vi "Chk_cre_dir.vi"(2 "error in (no error)":errorcluster, 3 "Path":path) -> (0 "error out":errorcluster, 1 "dup path":path)   [LabVIEW 2020]
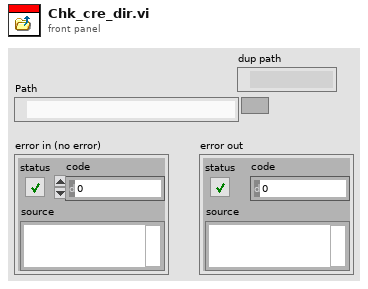
[diagram p1: front panel]
types:
  T1 = enum16{"open", "replace", "create", "open or create", "replace or create", "replace or create with confirmation"}
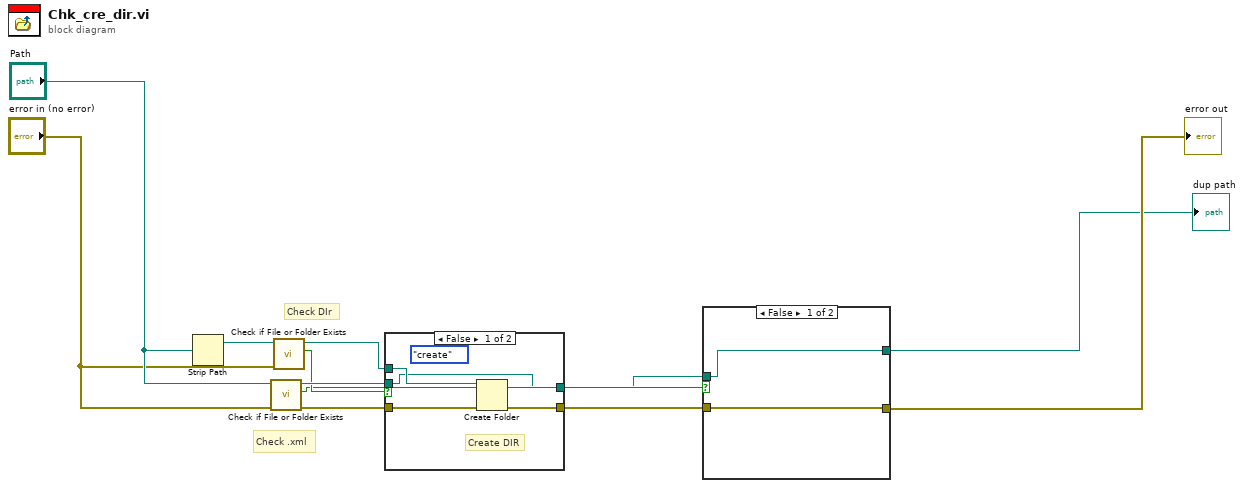
[diagram p0: block diagram]
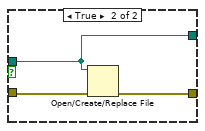
[diagram p2: hidden frame]
diagram:
  # "Check .xml"
  # "Check DIr"
  n1 = Strip Path(path="Path") -> (stripped path=w9:path)  [unwired: 1 out]
  n2 = call <vilib>:"Check if File or Folder Exists.vi"("error in (no error)"="error in (no error)", "path"="Path") -> ("error out"=w12:errorcluster, "file or folder exists?"=w5:bool, "dup path"=w11:path)  [unwired: 7 in]
  n3 = call <vilib>:"Check if File or Folder Exists.vi"("error in (no error)"="error in (no error)", "path"=w9) -> ("file or folder exists?"=w7:bool, "dup path"=w6:path)  [unwired: 7 in, 1 out]
  n4 = case shown="False" w7 {
    tunnel: w11 -> [w13 w17]
    tunnel: w12 -> [w16 w18]
    tunnel: [w15 w18] -> w4
    tunnel: [w13 w17] -> w2
    tunnel: w6 -> [w14 _]
    frame False {
      (unwired) T1."create" ("operation (0:open)")
      # "Create DIR"
      n5 = Create Folder(path (use dialog)=w14, error in=w16) -> (error out=w15:errorcluster)  [unwired: 1 in, 2 out]
    }
    frame True {
    }
  }
  n6 = case shown="False" w5 {
    tunnel: w2 -> [w19 w21]
    tunnel: w4 -> [w20 w23]
    tunnel: [w20 w22] -> w3
    tunnel: [w19 w21] -> w1
    frame False {
    }
    frame True {
      n7 = Open/Create/Replace File(file path (use dialog)=w21, error in=w23) -> (error out=w22:errorcluster)  [unwired: 4 in, 2 out]
    }
  }
  "error out" <- w3
  "dup path" <- w1
